vi "Compute Distance.vi"(8 "Y Image Resolution":i32, 9 "X Image Resolution":i32, 10 "Particle Scores":T1, 11 "Camera Type":enum16{"206", "1011"}(ring)) -> (1 "Center Target":bool, 2 "Target Center (-1 to 1)":cluster{"X":dbl, "Y":dbl}, 3 "Distance (ft)":dbl)   [LabVIEW 2013]
doc: "Using the camera lens information and the real world size of the target, use trig and simple math to determine the distance to the target. Also returns the location relative to the image center in a (-1 , 1) coordinate system that may be useful for steering the robot."
panel:
  in  "Camera view angle":dbl[](array[numeric])=[48.0, 47.0]
  # "Axis 206\nAxis M1011"
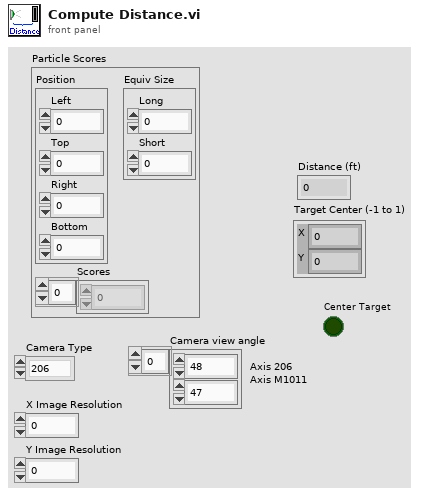
[diagram p1: front panel]
types:
  T1 = cluster{"Position":cluster{"Left":dbl, "Top":dbl, "Right":dbl, "Bottom":dbl}, "Scores":dbl[], "Equiv Size":cluster{"Long":dbl, "Short":dbl}}
  T2 = cluster{"X Image Resolution":i32, "Y Image Resolution":i32}
  T3 = cluster{"X Image Resolution":dbl, "Y Image Resolution":dbl}
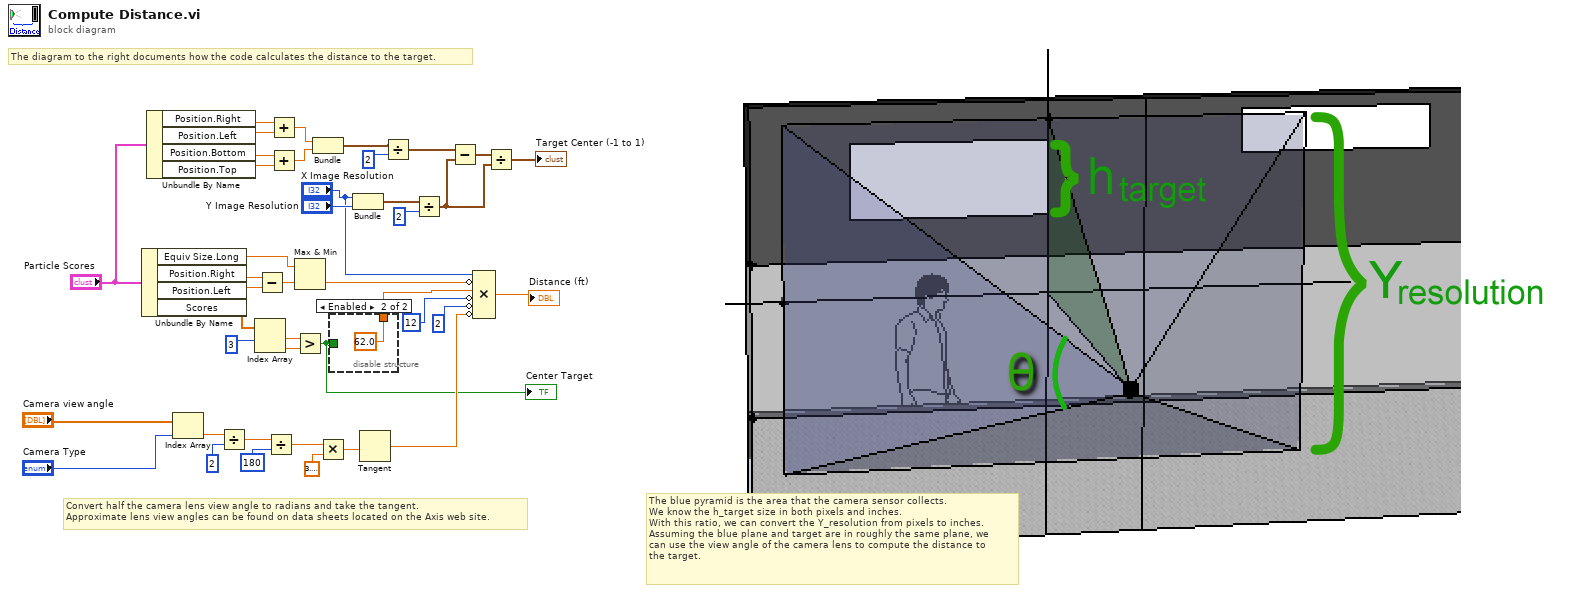
[diagram p0: block diagram]
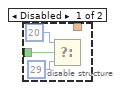
[diagram p2: hidden frame]
diagram:
  # "The blue pyramid is the area that the camera sensor collects.\nWe know the h_target size in both pixels and inches.\nWith this ratio, we can convert the Y_resolution from pixels to inches.\nAssuming the blue plane and target are in roughly the same plane, we\ncan use the view angle of the camera lens to compute the distance to\nthe target."
  # "Convert half the camera lens view angle to radians and take the tangent.\nApproximate lens view angles can be found on data sheets located on the Axis web site."
  # "The diagram to the right documents how the code calculates the distance to the target."
  n1 = Unbundle By Name("Particle Scores") -> ("Equiv Size.Long"=w6:dbl, "Position.Right"=w32:dbl, "Position.Left"=w31:dbl, "Scores"=w15:dbl[])
  n2 = Unbundle By Name("Particle Scores") -> ("Position.Right"=w26:dbl, "Position.Left"=w27:dbl, "Position.Bottom"=w29:dbl, "Position.Top"=w28:dbl)
  n3 = Index Array(array="Camera view angle", index="Camera Type") -> (element=w38:dbl)
  n4 = Divide(x=w38, y=2) -> (x/y=w35:dbl)
  n5 = Index Array(array=w15, index #1=3) -> (element #1=w8:dbl, element #2=w13:dbl)  [unwired: 1 in]
  n6 = Subtract(x=w32, y=w31) -> (x-y=w5:dbl)
  n7 = Divide(x=w35, y=180) -> (x/y=w34:dbl)
  n8 = Add(x=w26, y=w27) -> (x+y=w24:dbl)
  n9 = Add(x=w29, y=w28) -> (x+y=w23:dbl)
  n10 = Max & Min(x=w6, y=w5) -> (min(x,y)=w4:dbl)  [unwired: 1 out]
  n11 = Greater?(x=w8, y=w13) -> (0:w9:bool)
  "Center Target" <- w9
  n12 = Bundle(w24, w23) -> (w20:cluster{dbl, dbl})  [unwired: 1 in]
  n13 = Multiply(x=w34, y=3.141592653589793) -> (x*y=w36:dbl)
  n14 = disable-structure shown="Enabled" {
    disable-tunnel: w9 -> [w42 _]
    disable-tunnel: [_ 62.0 ("value")] -> w3
    frame Disabled {
      n15 = Select(t=20 ("Target Height (in)"), s=w42, f=29 ("Target Height (in)")) -> ()  [unwired: 1 out]
    }
    frame Enabled {
    }
  }
  n16 = Bundle("X Image Resolution"="X Image Resolution", "Y Image Resolution"="Y Image Resolution") -> (w22:T2)  [unwired: 1 in]
  n17 = Tangent(1:w36) -> (0:w12:dbl)
  n18 = Divide(x=w20, y=2) -> (x/y=w19:cluster{dbl, dbl})
  n19 = Divide(x=w22, y=2) -> (x/y=w17:T3)
  n20 = Subtract(x=w19, y=w17) -> (x-y=w18:cluster{dbl, dbl})
  n21 = Compound Arithmetic op=MULTIPLY("X Image Resolution", invert w4, w3, invert 12, invert 2, invert w12) -> (→"Distance (ft)":dbl)
  n22 = Divide(x=w18, y=w17) -> (x/y=→"Target Center (-1 to 1)":cluster{dbl, dbl})
